vi "Stop Module.vi"(6 "Timeout to Wait for Stop (s) (-1: no timeout)":dbl=-1.0, 8 "error in (no error)":errorcluster, 9 "Wait for Module to Stop? (F)":bool, 10 "Origin":string) -> (0 "error out":errorcluster)   [LabVIEW 2025, in "Data Logger v2.lvlib"]
doc: "Send the Stop request to the Module's Main.vi.\n\nIf <b>Wait for Module to Stop?</b> is TRUE, this VI will wait until the module main VI stops, and will timeout at the <b>Timeout to Wait for Stop</b> value. This value defaults to \"-1\", which means the VI will not timeout, and will always wait until the module main VI stops before completing execution.\n\nNote: The <b>Timeout to Wait for Stop</b> value is ignored if 'Wait for Module to Stop?' is set to FALSE.\n_____\nBased on Delacor QMH Project Template 3.1.0.34.\n\n<b>Note:</b> This VI was modified by the <b>Validate DQMH Module</b> tool so that it will still execute even on incoming error.\n\n<b>Note:</b> This VI was modified by the <b>Validate DQMH Module</b> tool to remove the Status Updated.vi subVI call."
uses:
  Data Logger v2.lvlib
  Stop Argument--cluster.ctl
  <vilib>/event_ctls.llb/usereventprio.ctl
panel:
  # "Note: The 'Timeout to Wait for Stop' value is ignored if 'Wait for Module to Stop?' is set to FALSE."
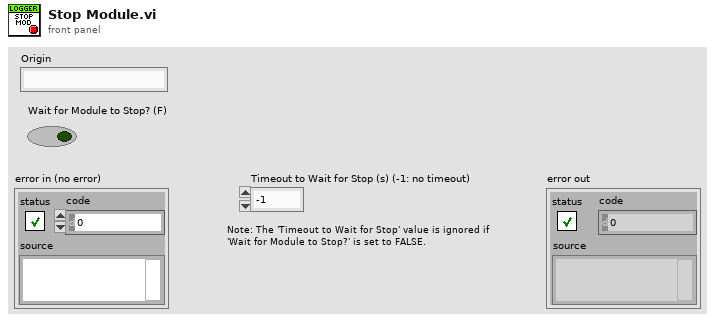
[diagram p1: front panel]
types:
  T1 = typedef "Data Logger v2.lvlib/Stop Argument--cluster.ctl" = cluster{"Origin":string, "Exit via Stop Module Req?":bool, "Wait for Module to stop?":bool}
  T2 = typedef "usereventprio.ctl" = enum32{"high priority", "normal priority"}
  T3 = typedef "Data Logger v2.lvlib/Request Events--cluster.ctl" = cluster{"Stop Module":refnum<user-event>, "Show Panel":refnum<user-event>, "Hide Panel":refnum<user-event>, "Get Module Execution Status":refnum<user-event>, "Show Diagram":refnum<user-event>, "Change Panel":refnum<user-event>, "Create New TDMS Log File":refnum<user-event>, "Write 2D Array to TDMS Log File":refnum<user-event>, "Close TDMS File":refnum<user-event>, "Write TDMS 2D String Array":refnum<user-event>, "Set Root Folder Path":refnum<user-event>, "Create New TDMS Log File (Relative Path)":refnum<user-event>, "Set Properties":refnum<user-event>}
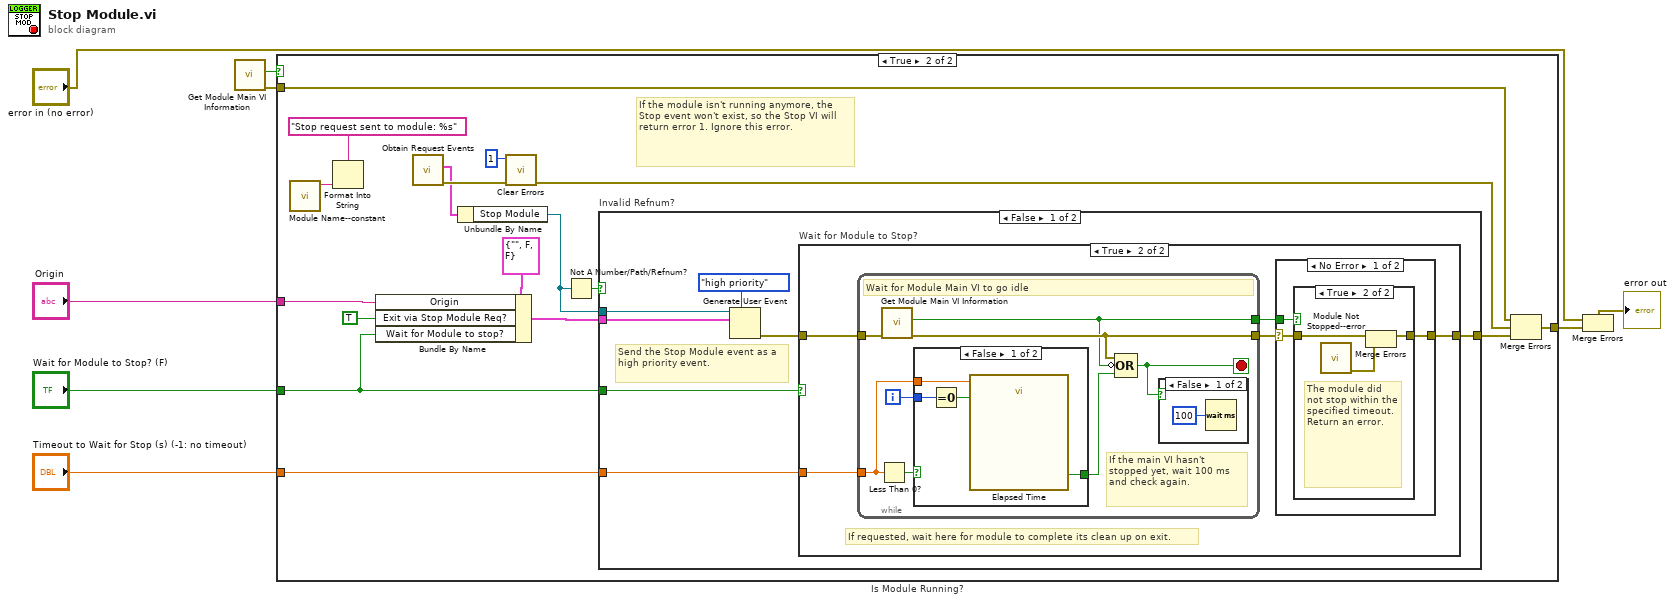
[diagram p0: block diagram]
diagram:
  n1 = call "Get Module Main VI Information.vi"() -> ("error out"=w5:errorcluster, "Is Module Running?"=w4:bool)  [unwired: 8 in, 2 out]
  n2 = case "Is Module Running?" shown="True" w4 {
    tunnel: [w9 w25] -> w8
    tunnel: "Origin" -> [_ w24]
    tunnel: w5 -> [w9 w14]
    tunnel: "Wait for Module to Stop? (F)" -> [_ w11]
    tunnel: "Timeout to Wait for Stop (s) (-1: no timeout)" -> [_ w10]
    frame False {
      # "The module is not running, there is no need to run the Stop Module code."
    }
    frame True {
      # "If the module isn't running anymore, the Stop event won't exist, so the Stop VI will return error 1. Ignore this error."
      n3 = call "Module Name--constant.vi"() -> ("Module Name"=w21:string)  [unwired: 11 in]
      n4 = Format Into String(format string="Stop request sent to module: %s", w21) -> ()  [unwired: 2 in, 2 out]
      n5 = Bundle By Name(cluster=T1 {"Origin"="", "Exit via Stop Module Req?"=FALSE, "Wait for Module to stop?"=FALSE} ("event data"), "Origin"=w24, "Exit via Stop Module Req?"=TRUE, "Wait for Module to stop?"=w11) -> (w17:T1)
      n6 = call "Obtain Request Events.vi"() -> ("error out"=w26:errorcluster, "Data Logger v2 Request Events"=w23:T3)  [unwired: 10 in]
      n7 = Unbundle By Name(w23) -> ("Stop Module"=w18:refnum<user-event>)
      n8 = call <vilib>:"Clear Errors.vi"("error in (no error)"=w26, "specific error code to clear (0: all)"=1) -> ("error out"=w13:errorcluster)  [unwired: 4 in, 1 out]
      n9 = Not A Number/Path/Refnum?(number/path/refnum=w18) -> (NaN/Path/Refnum?=w19:bool)
      n10 = case "Invalid Refnum?" shown="False" w19 {
        tunnel: [w28 _] -> w16
        tunnel: w18 -> [w33 _]
        tunnel: w17 -> [w31 _]
        tunnel: w11 -> [w29 _]
        tunnel: w10 -> [w27 _]
        frame False {
          # "Send the Stop Module event as a high priority event."
          n11 = Generate User Event(priority (normal)=usereventprio."high priority", user event=w33, event data cluster=w31) -> (error out=w30:errorcluster)  [unwired: 1 in, 1 out]
          n12 = case "Wait for Module to Stop?" shown="True" w29 {
            tunnel: w30 -> [w34 w38]
            tunnel: [w34 w36] -> w28
            tunnel: w27 -> [_ w39]
            frame False {
            }
            frame True {
              # "If requested, wait here for module to complete its clean up on exit."
              n13 = while {
                tunnel: w39 -> [w50]
                tunnel: w38 -> [w54]
                tunnel: [w53] -> w37
                tunnel: [w52] -> w35
                i -> [w55]
                stop <- w48 stop-if-true
                # "If the main VI hasn't stopped yet, wait 100 ms and check again."
                # "Wait for Module Main VI to go idle"
                n14 = Less Than 0?(x=w50) -> (x < 0?=w49:bool)
                n15 = call "Get Module Main VI Information.vi"("error in (no error)"=w54) -> ("error out"=w53:errorcluster, "Is Module Running?"=w52:bool)  [unwired: 7 in, 2 out]
                n16 = case shown="False" w49 {
                  tunnel: w50 -> [w57 _]
                  tunnel: w55 -> [w59 _]
                  tunnel: [w58 _] -> w51
                  frame False {
                    n17 = Equal To 0?(x=w59) -> (x = 0?=w60:bool)
                    n18 = call "Elapsed Time"("Time Target (s)"=w57, "Reset"=w60) -> ("Time has Elapsed"=w58:bool)  [unwired: 10 in, 7 out]
                  }
                  frame True {
                    # "User specified a timeout of -1, so don't keep track of the elapsed time since this loop started."
                  }
                }
                n19 = Compound Arithmetic op=OR(w53, invert w52, w51) -> (w48:bool)
                n20 = case shown="False" w48 {
                  frame False {
                    n21 = Wait (ms)(milliseconds to wait=u32 100) -> ()  [unwired: 1 out]
                  }
                  frame True {
                  }
                }
              }
              n22 = case shown="No Error" w37 {
                selector: w37 -> [w41 w47]
                tunnel: [w40 w47] -> w36
                tunnel: w35 -> [w42 _]
                frame No Error {
                  n23 = case shown="True" w42 {
                    tunnel: w41 -> [w43 w46]
                    tunnel: [w43 w45] -> w40
                    frame False {
                      # "The module stopped, and no error occurred."
                    }
                    frame True {
                      # "The module did not stop within the specified timeout. Return an error."
                      n24 = call "Module Not Stopped--error.vi"() -> ("error out"=w44:errorcluster)  [unwired: 11 in]
                      n25 = Merge Errors(w46, w44) -> (w45:errorcluster)
                    }
                  }
                }
                frame Error {
                  # "An error occurred while waiting for the module to stop. Return that error."
                }
              }
            }
          }
        }
        frame True {
          # "Module is exiting. No need to send the standard \"not running\" error that is sent in other request VIs."
        }
      }
      n26 = Merge Errors(w14, w13, w16) -> (w25:errorcluster)
    }
  }
  n27 = Merge Errors("error in (no error)", w8) -> (→"error out":errorcluster)
